vi "WPI_RobotDriveMotors.vi"(0 "RobotDriveDevRef":string, 7 "LeftSpeed":dbl, 11 "RightSpeed":dbl) -> (4 "RobotDriveDevRef":string, 15 "MotorValues":dbl)   [LabVIEW 2017]
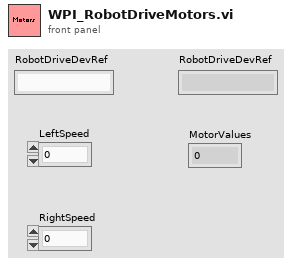
[diagram p1: front panel]
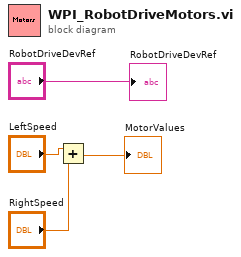
[diagram p0: block diagram]
diagram:
  n1 = Add(x="LeftSpeed", y="RightSpeed") -> (x+y=→"MotorValues":dbl)
  "RobotDriveDevRef" <- "RobotDriveDevRef"
